vi "Control AlgorithmV3.vi"(5 "Gear (H/L)":bool, 6 "PID Gains":cluster{"P":dbl, "I":dbl, "D":dbl}, 7 "Init":bool, 8 "Motor to Control":u8, 9 "Manual Control":bool, 10 "Wheel Angles":dbl[](array[numeric]), 11 "JoystickIn":i32[](array[slide]) scale=-37626.0..37626.0) -> (2 "Target Angles":dbl[](array[numeric]), 3 "MotorsOut":u16[](array[slide]) scale=0.0..512.0)   [LabVIEW 2013, in "ProcessorHelperFunctions.lvlib"]
uses:
  ProcessorHelperFunctions.lvlib
panel:
  out "AglErr4":dbl
  out "AglErr3":dbl
  out "AglErr2":dbl
  out "AglErr1":dbl
  in  "SteeringAssist4_H":dbl=-0.5 format="%#_13g"
  in  "SteeringAssist3_H":dbl=-0.5 format="%#_13g"
  in  "SteeringAssist2_H":dbl=-0.7 format="%#_13g"
  in  "SteeringAssist1_H":dbl=-0.5 format="%#_13g"
  in  "SteeringAssist4_L":dbl=-0.4 format="%#_13g"
  in  "SteeringAssist3_L":dbl=-0.3 format="%#_13g"
  in  "SteeringAssist2_L":dbl=-0.5 format="%#_13g"
  in  "SteeringAssist1_L":dbl=-0.5 format="%#_13g"
  out "JoystickIn_DB":i32[](array[slide]) scale=-37626.0..37626.0
  out "y":dbl
  out "x":dbl
  out "Point":picture
  out "ReverseDir?4":bool
  out "ReverseDir?3":bool
  out "ReverseDir?2":bool
  out "ReverseDir?1":bool
  out "Radius1":dbl
  out "Radius2":dbl
  out "Radius3":dbl
  out "Radius4":dbl
  in  "RJoyMagGain":dbl=0.6
  in  "LJoyMagGain":dbl=1.0
  out "OldAngle4":dbl
  out "OldAngle3":dbl
  out "OldAngle2":dbl
  out "OldAngle1":dbl
  in  "Yw":dbl=15.5
  in  "Xw":dbl=21.5
  # "Xw is x distance between the\nwheels on the robot"
  # "------------------------------------ LOCAL VARIABLES ---------------------------------------"
  # "Yw is y distance between the\nwheels on the robot"
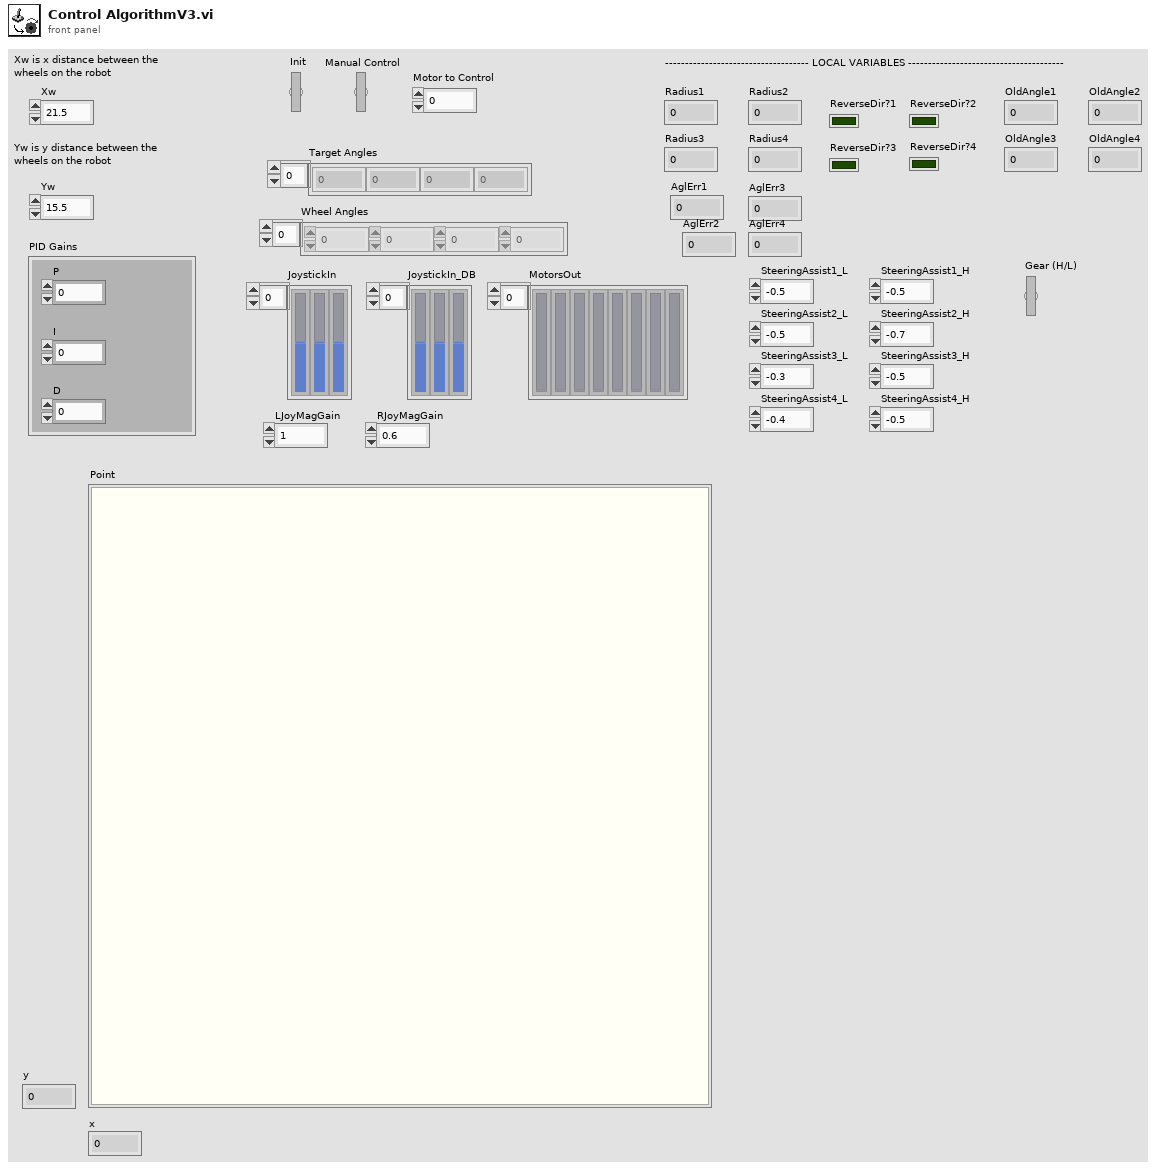
[diagram p1: front panel]
types:
  T1 = cluster{"Width":u16, "Style":enum32{"Solid", "Dash", "Dot", "DashDot", "DashDotDot"}}
  T2 = cluster{"JoystickOut[0]":i32, "JoystickOut[1]":i32, "JoystickOut[2]":i32, "JoystickOut[3]":i32, "JoystickOut[4]":i32, "JoystickOut[5]":i32, "JoystickOut[6]":i32, "JoystickOut[7]":i32, "JoystickOut[8]":i32}
  T3 = cluster{"Wheel Angles[0]":dbl, "Wheel Angles[1]":dbl, "Wheel Angles[2]":dbl, "Wheel Angles[3]":dbl, "Wheel Angles[4]":dbl, "Wheel Angles[5]":dbl, "Wheel Angles[6]":dbl, "Wheel Angles[7]":dbl, "Wheel Angles[8]":dbl}
  T4 = cluster{"[0]":dbl, "[1]":dbl, "[2]":dbl, "[3]":dbl, "[4]":dbl, "[5]":dbl, "[6]":dbl, "[7]":dbl, "[8]":dbl}
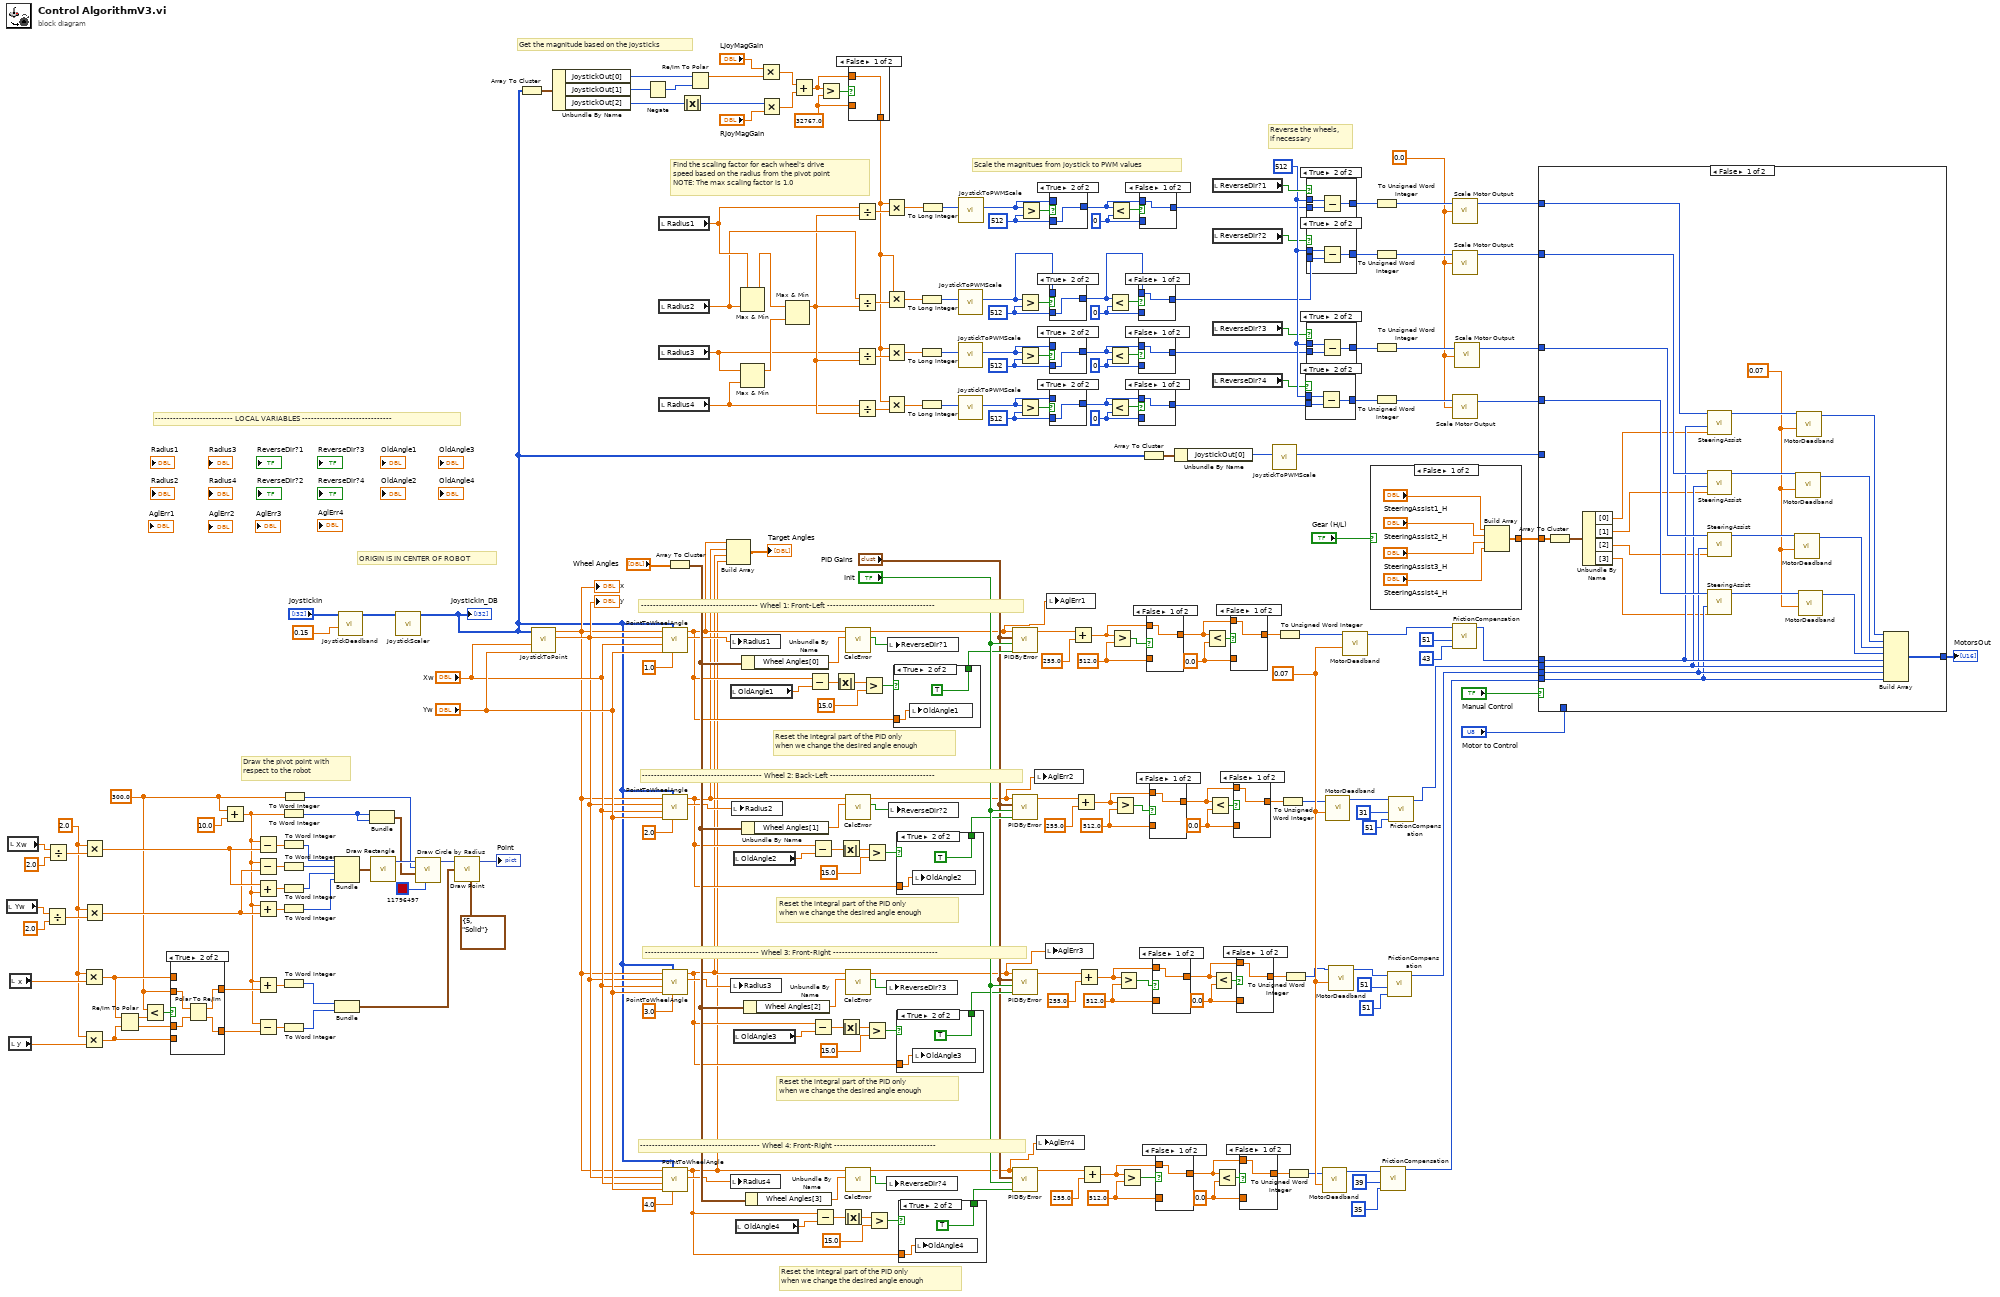
[diagram p0: block diagram]
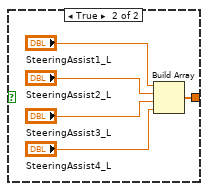
[diagram p2: hidden frame]
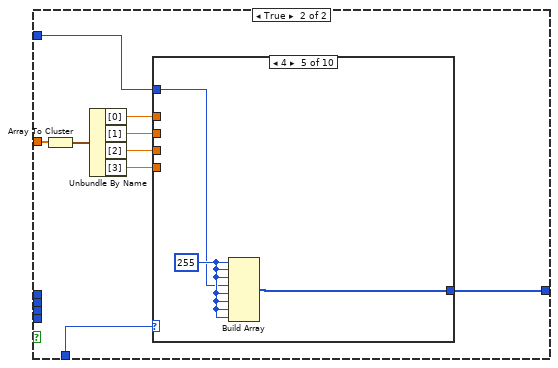
[diagram p17: hidden frame]
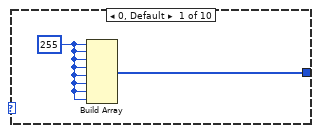
[diagram p18: hidden frame]
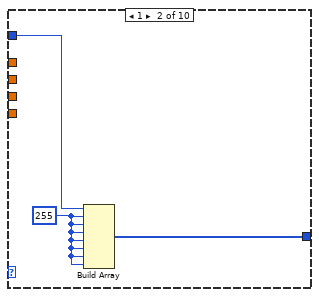
[diagram p19: hidden frame]
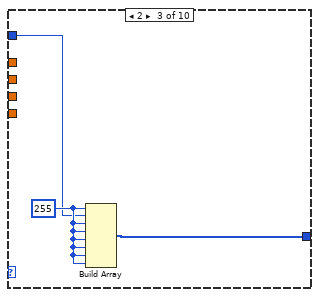
[diagram p20: hidden frame]
diagram:
  w1 = 0.0
  w32 = 0.07 ("DBPercent")
  w42 = 32767.0 ("y")
  w50 = 0 ("y")
  w51 = 512 ("y")
  w61 = 0 ("y")
  w60 = 512 ("y")
  w68 = 0 ("y")
  w69 = 512 ("y")
  w83 = u16 512 ("x")
  w114 = 2.0 ("x")
  w95 = 300.0 ("x")
  w165 = 0 ("y")
  w164 = 512 ("y")
  w184 = 0.0 ("y")
  w182 = 512.0 ("y")
  w190 = 0.0 ("y")
  w192 = 512.0 ("y")
  w200 = 0.0 ("y")
  w198 = 512.0 ("y")
  w205 = 0.0 ("y")
  w207 = 512.0 ("y")
  # "Scale the magnitues from joystick to PWM values"
  # "Get the magnitude based on the joysticks"
  # "Reverse the wheels,\nif necessary"
  # "Draw the pivot point with\nrespect to the robot"
  # "Find the scaling factor for each wheel's drive\nspeed based on the radius from the pivot point\nNOTE: The max scaling factor is 1.0"
  # "Reset the integral part of the PID only\nwhen we change the desired angle enough"
  # "Reset the integral part of the PID only\nwhen we change the desired angle enough"
  # "Reset the integral part of the PID only\nwhen we change the desired angle enough"
  # "Reset the integral part of the PID only\nwhen we change the desired angle enough"
  # "-------------------------- LOCAL VARIABLES ------------------------------"
  # "---------------------------------------- Wheel 4: Front-Right ----------------------------------"
  # "-------------------------------------- Wheel 3: Front-Right -----------------------------------"
  # "---------------------------------------- Wheel 2: Back-Left -----------------------------------"
  # "--------------------------------------- Wheel 1: Front-Left ------------------------------------"
  # "ORIGIN IS IN CENTER OF ROBOT"
  n1 = local read "Yw"() -> (w139:dbl)
  n2 = local read "Xw"() -> (w142:dbl)
  n3 = local read "y"() -> (w115:dbl)
  n4 = local read "x"() -> (w122:dbl)
  n5 = Divide(x=w139, y=2.0) -> (x/y=w119:dbl)
  n6 = Divide(x=w142, y=2.0) -> (x/y=w120:dbl)
  n7 = Multiply(x=w114, y=w122) -> (x*y=w109:dbl)
  n8 = Multiply(x=w114, y=w115) -> (x*y=w108:dbl)
  n9 = Multiply(x=w114, y=w120) -> (x*y=w117:dbl)
  n10 = Multiply(x=w114, y=w119) -> (x*y=w116:dbl)
  n11 = Re/Im To Polar(2:w108, 3:w109) -> (0:w107:dbl, 1:w111:dbl)
  n12 = Less?(x=w95, y=w111) -> (x < y?=w110:bool)
  n13 = case shown="True" w110 {
    tunnel: w109 -> [w251 _]
    tunnel: w108 -> [w250 _]
    tunnel: w95 -> [_ w255]
    tunnel: w107 -> [_ w254]
    tunnel: [w251 w253] -> w105
    tunnel: [w250 w252] -> w106
    frame False {
    }
    frame True {
      n14 = Polar To Re/Im(2:w254, 3:w255) -> (0:w252:dbl, 1:w253:dbl)
    }
  }
  n15 = Add(x=w95, y=10.0) -> (x+y=w94:dbl)
  n16 = Subtract(x=w94, y=w117) -> (x-y=w100:dbl)
  n17 = Subtract(x=w94, y=w116) -> (x-y=w129:dbl)
  n18 = Add(x=w117, y=w94) -> (x+y=w128:dbl)
  n19 = Add(x=w94, y=w116) -> (x+y=w127:dbl)
  n20 = Add(x=w94, y=w105) -> (x+y=w104:dbl)
  n21 = Subtract(x=w94, y=w106) -> (x-y=w103:dbl)
  n22 = To Word Integer(number=w94) -> (16bit integer=w93:i16)
  n23 = To Word Integer(number=w100) -> (16bit integer=w130:i16)
  n24 = To Word Integer(number=w129) -> (16bit integer=w126:i16)
  n25 = To Word Integer(number=w128) -> (16bit integer=w125:i16)
  n26 = To Word Integer(number=w127) -> (16bit integer=w124:i16)
  n27 = To Word Integer(number=w104) -> (16bit integer=w138:i16)
  n28 = To Word Integer(number=w103) -> (16bit integer=w137:i16)
  n29 = To Word Integer(number=w95) -> (16bit integer=w97:i16)
  n30 = Bundle(w130, w126, w125, w124) -> (w123:cluster{i16, i16, i16, i16})  [unwired: 1 in]
  n31 = Bundle(w138, w137) -> (w136:cluster{i16, i16})  [unwired: 1 in]
  n32 = call "JoystickDeadband.vi"("DBPercent"=0.15, "JoystickIn"="JoystickIn") -> ("JoystickOut"=w2:i32[])  [unwired: 9 in]
  n33 = Bundle(w93, w93) -> (w99:cluster{i16, i16})  [unwired: 1 in]
  n34 = call <vilib>:"Draw Rectangle.vi"("rect"=w123) -> ("new picture"=w102:picture)  [unwired: 8 in]
  n35 = call "JoystickScaler.vi"("JoystickIn"=w2) -> ("JoystickOut"=w3:i32[])  [unwired: 10 in]
  "JoystickIn_DB" <- w3
  n36 = call <vilib>:"Draw Circle by Radius.vi"("color(black)"=u32 11796497, "pixel center"=w99, "radius"=w97, "picture"=w102) -> ("new picture"=w101:picture)  [unwired: 7 in]
  n37 = call <vilib>:"Draw Point.vi"("picture"=w101, "point(x,y)"=w136, "pen"=T1 {"Width"=5, "Style"=enum."Solid"}) -> ("new picture"=→"Point":picture)  [unwired: 6 in]
  n38 = Array To Cluster(array=w3) -> (cluster=w176:T2)
  n39 = call "JoystickToPoint.vi"("Yw"="Yw", "Xw"="Xw", "JoystickIn"=w3) -> ("y"=w243:dbl, "x"=w242:dbl)  [unwired: 7 in]
  "x" <- w242
  "y" <- w243
  n40 = Unbundle By Name(w176) -> ("JoystickOut[0]"=w175:i32, "JoystickOut[1]"=w174:i32, "JoystickOut[2]"=w171:i32)
  n41 = Negate(x=w174) -> (-x=w118:i32)
  n42 = local read "Radius1"() -> (w151:dbl)
  n43 = local read "Radius2"() -> (w150:dbl)
  n44 = local read "Radius3"() -> (w148:dbl)
  n45 = local read "Radius4"() -> (w147:dbl)
  n46 = call "PointToWheelAngle.vi"("Wheel Number"=1.0, "JoystickIn"=w3, "Yw"="Yw", "Xw"="Xw", "y"=w243, "x"=w242) -> ("Radius"=w161:dbl, "Desired Angle"=w92:dbl)  [unwired: 4 in]
  n47 = call "PointToWheelAngle.vi"("Wheel Number"=2.0, "JoystickIn"=w3, "Yw"="Yw", "Xw"="Xw", "y"=w243, "x"=w242) -> ("Radius"=w160:dbl, "Desired Angle"=w91:dbl)  [unwired: 4 in]
  n48 = call "PointToWheelAngle.vi"("Wheel Number"=3.0, "JoystickIn"=w3, "Yw"="Yw", "Xw"="Xw", "y"=w243, "x"=w242) -> ("Radius"=w159:dbl, "Desired Angle"=w90:dbl)  [unwired: 4 in]
  n49 = call "PointToWheelAngle.vi"("Wheel Number"=4.0, "JoystickIn"=w3, "Yw"="Yw", "Xw"="Xw", "y"=w243, "x"=w242) -> ("Radius"=w158:dbl, "Desired Angle"=w89:dbl)  [unwired: 4 in]
  n50 = Array To Cluster(array="Wheel Angles") -> (cluster=w240:T3)
  n51 = Absolute Value(x=w171) -> (abs(x)=w45:i32)
  n52 = Re/Im To Polar(2:w118, 3:w175) -> (1:w173:dbl)  [unwired: 1 out]
  n53 = Build Array(w92, w91, w90, w89) -> (→"Target Angles":dbl[])
  n54 = local write "Radius1"(w161) -> ()
  n55 = local read "OldAngle1"() -> (w235:dbl)
  n56 = local write "Radius4"(w158) -> ()
  n57 = local write "Radius3"(w159) -> ()
  n58 = local write "Radius2"(w160) -> ()
  n59 = local read "OldAngle2"() -> (w228:dbl)
  n60 = local read "OldAngle3"() -> (w223:dbl)
  n61 = local read "OldAngle4"() -> (w218:dbl)
  n62 = Max & Min(x=w151, y=w150) -> (max(x,y)=w153:dbl)  [unwired: 1 out]
  n63 = Max & Min(x=w148, y=w147) -> (max(x,y)=w152:dbl)  [unwired: 1 out]
  n64 = Unbundle By Name(w240) -> ("Wheel Angles[0]"=w239:dbl)
  n65 = Unbundle By Name(w240) -> ("Wheel Angles[1]"=w238:dbl)
  n66 = Unbundle By Name(w240) -> ("Wheel Angles[2]"=w237:dbl)
  n67 = Unbundle By Name(w240) -> ("Wheel Angles[3]"=w236:dbl)
  n68 = Multiply(x="LJoyMagGain", y=w173) -> (x*y=w169:dbl)
  n69 = Multiply(x=w45, y="RJoyMagGain") -> (x*y=w168:dbl)
  n70 = Max & Min(x=w153, y=w152) -> (max(x,y)=w149:dbl)  [unwired: 1 out]
  n71 = Add(x=w169, y=w168) -> (x+y=w43:dbl)
  n72 = Subtract(x=w92, y=w235) -> (x-y=w234:dbl)
  n73 = Subtract(x=w91, y=w228) -> (x-y=w227:dbl)
  n74 = Subtract(x=w90, y=w223) -> (x-y=w222:dbl)
  n75 = Subtract(x=w89, y=w218) -> (x-y=w217:dbl)
  n76 = Greater?(x=w43, y=w42) -> (0:w44:bool)
  n77 = Absolute Value(x=w234) -> (abs(x)=w233:dbl)
  n78 = Absolute Value(x=w227) -> (abs(x)=w226:dbl)
  n79 = Absolute Value(x=w222) -> (abs(x)=w221:dbl)
  n80 = Absolute Value(x=w217) -> (abs(x)=w216:dbl)
  n81 = call "CalcError.vi"("Actual Angle"=w239, "Desired Angle"=w92) -> ("ReverseDir?"=w157:bool, "Angle Error"=w15:dbl)  [unwired: 8 in]
  n82 = call "CalcError.vi"("Actual Angle"=w238, "Desired Angle"=w91) -> ("ReverseDir?"=w156:bool, "Angle Error"=w14:dbl)  [unwired: 8 in]
  n83 = call "CalcError.vi"("Actual Angle"=w237, "Desired Angle"=w90) -> ("ReverseDir?"=w155:bool, "Angle Error"=w13:dbl)  [unwired: 8 in]
  n84 = call "CalcError.vi"("Actual Angle"=w236, "Desired Angle"=w89) -> ("ReverseDir?"=w154:bool, "Angle Error"=w12:dbl)  [unwired: 8 in]
  n85 = case shown="False" w44 {
    tunnel: w43 -> [w256 _]
    tunnel: w42 -> [_ w257]
    tunnel: [w256 w257] -> w33
    frame False {
    }
    frame True {
    }
  }
  n86 = Divide(x=w151, y=w149) -> (x/y=w78:dbl)
  n87 = Divide(x=w150, y=w149) -> (x/y=w77:dbl)
  n88 = Divide(x=w148, y=w149) -> (x/y=w76:dbl)
  n89 = Divide(x=w147, y=w149) -> (x/y=w75:dbl)
  n90 = Greater?(x=w233, y=15.0) -> (0:w231:bool)
  n91 = Greater?(x=w226, y=15.0) -> (0:w224:bool)
  n92 = Greater?(x=w221, y=15.0) -> (0:w219:bool)
  n93 = Greater?(x=w216, y=15.0) -> (0:w214:bool)
  n94 = Multiply(x=w33, y=w78) -> (x*y=w74:dbl)
  n95 = Multiply(x=w33, y=w77) -> (x*y=w65:dbl)
  n96 = Multiply(x=w33, y=w76) -> (x*y=w56:dbl)
  n97 = Multiply(x=w33, y=w75) -> (x*y=w47:dbl)
  n98 = local write "ReverseDir?3"(w155) -> ()
  n99 = local write "ReverseDir?4"(w154) -> ()
  n100 = local write "ReverseDir?1"(w157) -> ()
  n101 = local write "ReverseDir?2"(w156) -> ()
  n102 = case shown="True" w231 {
    tunnel: w92 -> [_ w260]
    tunnel: [FALSE ("Reset1") TRUE ("Reset1")] -> w229
    frame False {
    }
    frame True {
      n103 = local write "OldAngle1"(w260) -> ()
    }
  }
  n104 = case shown="True" w224 {
    tunnel: w91 -> [_ w263]
    tunnel: [FALSE ("Reset1") TRUE ("Reset1")] -> w211
    frame False {
    }
    frame True {
      n105 = local write "OldAngle2"(w263) -> ()
    }
  }
  n106 = case shown="True" w219 {
    tunnel: w90 -> [_ w266]
    tunnel: [FALSE ("Reset1") TRUE ("Reset1")] -> w213
    frame False {
    }
    frame True {
      n107 = local write "OldAngle3"(w266) -> ()
    }
  }
  n108 = case shown="True" w214 {
    tunnel: w89 -> [_ w269]
    tunnel: [FALSE ("Reset1") TRUE ("Reset1")] -> w212
    frame False {
    }
    frame True {
      n109 = local write "OldAngle4"(w269) -> ()
    }
  }
  n110 = To Long Integer(number=w65) -> (32bit integer=w66:i32)
  n111 = To Long Integer(number=w56) -> (32bit integer=w63:i32)
  n112 = To Long Integer(number=w47) -> (32bit integer=w48:i32)
  n113 = To Long Integer(number=w74) -> (32bit integer=w167:i32)
  n114 = call "JoystickToPWMScale.vi"("Numeric"=w66) -> ("Numeric 2"=w71:u16)  [unwired: 10 in]
  n115 = call "JoystickToPWMScale.vi"("Numeric"=w63) -> ("Numeric 2"=w58:u16)  [unwired: 10 in]
  n116 = call "JoystickToPWMScale.vi"("Numeric"=w48) -> ("Numeric 2"=w53:u16)  [unwired: 10 in]
  n117 = call "JoystickToPWMScale.vi"("Numeric"=w167) -> ("Numeric 2"=w162:u16)  [unwired: 10 in]
  n118 = call "PIDByError.vi"("Error"=w15, "PID Gains"="PID Gains", "Init"="Init", "Reset"=w229) -> ("Control"=w210:dbl)  [unwired: 6 in]
  n119 = call "PIDByError.vi"("Error"=w14, "PID Gains"="PID Gains", "Init"="Init", "Reset"=w211) -> ("Control"=w195:dbl)  [unwired: 6 in]
  n120 = call "PIDByError.vi"("Error"=w13, "PID Gains"="PID Gains", "Init"="Init", "Reset"=w213) -> ("Control"=w187:dbl)  [unwired: 6 in]
  n121 = call "PIDByError.vi"("Error"=w12, "PID Gains"="PID Gains", "Init"="Init", "Reset"=w212) -> ("Control"=w179:dbl)  [unwired: 6 in]
  n122 = Greater?(x=w71, y=w69) -> (0:w70:bool)
  n123 = Greater?(x=w58, y=w60) -> (0:w59:bool)
  n124 = Greater?(x=w53, y=w51) -> (0:w52:bool)
  n125 = Greater?(x=w162, y=w164) -> (0:w163:bool)
  n126 = local write "AglErr2"(w14) -> ()
  n127 = local write "AglErr4"(w12) -> ()
  n128 = local write "AglErr3"(w13) -> ()
  n129 = local write "AglErr1"(w15) -> ()
  n130 = case shown="True" w70 {
    tunnel: w69 -> [_ w271]
    tunnel: w71 -> [w270 _]
    tunnel: [w270 w271] -> w67
    frame False {
    }
    frame True {
    }
  }
  n131 = case shown="True" w59 {
    tunnel: w60 -> [_ w273]
    tunnel: w58 -> [w272 _]
    tunnel: [w272 w273] -> w62
    frame False {
    }
    frame True {
    }
  }
  n132 = case shown="True" w52 {
    tunnel: w51 -> [_ w275]
    tunnel: w53 -> [w274 _]
    tunnel: [w274 w275] -> w49
    frame False {
    }
    frame True {
    }
  }
  n133 = case shown="True" w163 {
    tunnel: w164 -> [_ w277]
    tunnel: w162 -> [w276 _]
    tunnel: [w276 w277] -> w166
    frame False {
    }
    frame True {
    }
  }
  n134 = Add(x=w210, y=255.0) -> (x+y=w206:dbl)
  n135 = Add(x=w195, y=255.0) -> (x+y=w199:dbl)
  n136 = Add(x=w187, y=255.0) -> (x+y=w191:dbl)
  n137 = Add(x=w179, y=255.0) -> (x+y=w183:dbl)
  n138 = Less?(x=w67, y=w68) -> (x < y?=w72:bool)
  n139 = Less?(x=w62, y=w61) -> (x < y?=w57:bool)
  n140 = Less?(x=w49, y=w50) -> (x < y?=w54:bool)
  n141 = Less?(x=w166, y=w165) -> (x < y?=w131:bool)
  n142 = Greater?(x=w206, y=w207) -> (0:w208:bool)
  n143 = Greater?(x=w199, y=w198) -> (0:w197:bool)
  n144 = Greater?(x=w191, y=w192) -> (0:w193:bool)
  n145 = Greater?(x=w183, y=w182) -> (0:w181:bool)
  n146 = case shown="False" w72 {
    tunnel: w68 -> [_ w279]
    tunnel: w67 -> [w278 _]
    tunnel: [w278 w279] -> w64
    frame False {
    }
    frame True {
    }
  }
  n147 = case shown="False" w57 {
    tunnel: w61 -> [_ w281]
    tunnel: w62 -> [w280 _]
    tunnel: [w280 w281] -> w55
    frame False {
    }
    frame True {
    }
  }
  n148 = case shown="False" w54 {
    tunnel: w50 -> [_ w283]
    tunnel: w49 -> [w282 _]
    tunnel: [w282 w283] -> w46
    frame False {
    }
    frame True {
    }
  }
  n149 = case shown="False" w131 {
    tunnel: w165 -> [_ w285]
    tunnel: w166 -> [w284 _]
    tunnel: [w284 w285] -> w73
    frame False {
    }
    frame True {
    }
  }
  n150 = Array To Cluster(array=w3) -> (cluster=w146:T2)
  n151 = case shown="False" w208 {
    tunnel: w207 -> [_ w287]
    tunnel: w206 -> [w286 _]
    tunnel: [w286 w287] -> w204
    frame False {
    }
    frame True {
    }
  }
  n152 = case shown="False" w197 {
    tunnel: w198 -> [_ w289]
    tunnel: w199 -> [w288 _]
    tunnel: [w288 w289] -> w201
    frame False {
    }
    frame True {
    }
  }
  n153 = case shown="False" w193 {
    tunnel: w192 -> [_ w291]
    tunnel: w191 -> [w290 _]
    tunnel: [w290 w291] -> w189
    frame False {
    }
    frame True {
    }
  }
  n154 = case shown="False" w181 {
    tunnel: w182 -> [_ w293]
    tunnel: w183 -> [w292 _]
    tunnel: [w292 w293] -> w185
    frame False {
    }
    frame True {
    }
  }
  n155 = Unbundle By Name(w146) -> ("JoystickOut[0]"=w145:i32)
  n156 = Less?(x=w204, y=w205) -> (x < y?=w132:bool)
  n157 = Less?(x=w201, y=w200) -> (x < y?=w133:bool)
  n158 = Less?(x=w189, y=w190) -> (x < y?=w134:bool)
  n159 = local read "ReverseDir?1"() -> (w87:bool)
  n160 = local read "ReverseDir?2"() -> (w81:bool)
  n161 = local read "ReverseDir?3"() -> (w80:bool)
  n162 = local read "ReverseDir?4"() -> (w79:bool)
  n163 = Less?(x=w185, y=w184) -> (x < y?=w135:bool)
  n164 = case shown="False" w132 {
    tunnel: w205 -> [_ w295]
    tunnel: w204 -> [w294 _]
    tunnel: [w294 w295] -> w203
    frame False {
    }
    frame True {
    }
  }
  n165 = case shown="False" w133 {
    tunnel: w200 -> [_ w297]
    tunnel: w201 -> [w296 _]
    tunnel: [w296 w297] -> w202
    frame False {
    }
    frame True {
    }
  }
  n166 = case shown="False" w134 {
    tunnel: w190 -> [_ w299]
    tunnel: w189 -> [w298 _]
    tunnel: [w298 w299] -> w188
    frame False {
    }
    frame True {
    }
  }
  n167 = case shown="False" w135 {
    tunnel: w184 -> [_ w301]
    tunnel: w185 -> [w300 _]
    tunnel: [w300 w301] -> w186
    frame False {
    }
    frame True {
    }
  }
  n168 = call "JoystickToPWMScale.vi"("Numeric"=w145) -> ("Numeric 2"=w144:u16)  [unwired: 10 in]
  n169 = To Unsigned Word Integer(number=w203) -> (unsigned 16bit integer=w23:u16)
  n170 = To Unsigned Word Integer(number=w202) -> (unsigned 16bit integer=w21:u16)
  n171 = To Unsigned Word Integer(number=w188) -> (unsigned 16bit integer=w19:u16)
  n172 = To Unsigned Word Integer(number=w186) -> (unsigned 16bit integer=w17:u16)
  n173 = case shown="True" w79 {
    tunnel: w46 -> [w302 w305]
    tunnel: w83 -> [_ w304]
    tunnel: [w302 w303] -> w82
    frame False {
    }
    frame True {
      n174 = Subtract(x=w304, y=w305) -> (x-y=w303:i32)
    }
  }
  n175 = case shown="True" w87 {
    tunnel: w73 -> [w306 w309]
    tunnel: w83 -> [_ w308]
    tunnel: [w306 w307] -> w86
    frame False {
    }
    frame True {
      n176 = Subtract(x=w308, y=w309) -> (x-y=w307:i32)
    }
  }
  n177 = case shown="True" w81 {
    tunnel: w64 -> [w310 w313]
    tunnel: w83 -> [_ w312]
    tunnel: [w310 w311] -> w84
    frame False {
    }
    frame True {
      n178 = Subtract(x=w312, y=w313) -> (x-y=w311:i32)
    }
  }
  n179 = case shown="True" w80 {
    tunnel: w55 -> [w314 w317]
    tunnel: w83 -> [_ w316]
    tunnel: [w314 w315] -> w85
    frame False {
    }
    frame True {
      n180 = Subtract(x=w316, y=w317) -> (x-y=w315:i32)
    }
  }
  n181 = call "MotorDeadband.vi"("DBPercent"=w32, "MotorIn"=w17) -> ("MotorOut"=w16:u16)  [unwired: 9 in]
  n182 = call "MotorDeadband.vi"("DBPercent"=w32, "MotorIn"=w21) -> ("MotorOut"=w20:u16)  [unwired: 9 in]
  n183 = call "MotorDeadband.vi"("DBPercent"=w32, "MotorIn"=w19) -> ("MotorOut"=w18:u16)  [unwired: 9 in]
  n184 = call "MotorDeadband.vi"("DBPercent"=w32, "MotorIn"=w23) -> ("MotorOut"=w22:u16)  [unwired: 9 in]
  n185 = case shown="False" "Gear (H/L)" {
    tunnel: [w318 w323] -> w29
    frame False {
      n186 = Build Array("SteeringAssist1_H", "SteeringAssist2_H", "SteeringAssist3_H", "SteeringAssist4_H") -> (w318:dbl[])
    }
    frame True {
      n187 = Build Array("SteeringAssist1_L", "SteeringAssist2_L", "SteeringAssist3_L", "SteeringAssist4_L") -> (w323:dbl[])
    }
  }
  n188 = To Unsigned Word Integer(number=w86) -> (unsigned 16bit integer=w11:u16)
  n189 = To Unsigned Word Integer(number=w84) -> (unsigned 16bit integer=w10:u16)
  n190 = To Unsigned Word Integer(number=w85) -> (unsigned 16bit integer=w9:u16)
  n191 = To Unsigned Word Integer(number=w82) -> (unsigned 16bit integer=w8:u16)
  n192 = call "FrictionCompensation.vi"("REV Compensation"=u16 35, "FWD Compensation"=u16 39, "Input"=w16) -> ("Output"=w24:u16)  [unwired: 8 in]
  n193 = call "FrictionCompensation.vi"("REV Compensation"=u16 51, "FWD Compensation"=u16 51, "Input"=w18) -> ("Output"=w25:u16)  [unwired: 8 in]
  n194 = call "FrictionCompensation.vi"("REV Compensation"=u16 51, "FWD Compensation"=u16 31, "Input"=w20) -> ("Output"=w26:u16)  [unwired: 8 in]
  n195 = call "FrictionCompensation.vi"("REV Compensation"=u16 43, "FWD Compensation"=u16 51, "Input"=w22) -> ("Output"=w27:u16)  [unwired: 8 in]
  n196 = call "Scale Motor Output.vi"("Error Input"=w1, "Motor Input"=w11) -> ("Output"=w7:u16)  [unwired: 1 in]
  n197 = call "Scale Motor Output.vi"("Error Input"=w1, "Motor Input"=w10) -> ("Output"=w6:u16)  [unwired: 1 in]
  n198 = call "Scale Motor Output.vi"("Error Input"=w1, "Motor Input"=w8) -> ("Output"=w4:u16)  [unwired: 1 in]
  n199 = call "Scale Motor Output.vi"("Error Input"=w1, "Motor Input"=w9) -> ("Output"=w5:u16)  [unwired: 1 in]
  n200 = case shown="False" "Manual Control" {
    tunnel: w27 -> [w346 _]
    tunnel: w26 -> [w345 _]
    tunnel: w25 -> [w344 _]
    tunnel: w24 -> [w343 _]
    tunnel: [w351 w358] -> w30
    tunnel: "Motor to Control" -> [_ w360]
    tunnel: w7 -> [w350 _]
    tunnel: w6 -> [w349 _]
    tunnel: w5 -> [w348 _]
    tunnel: w4 -> [w347 _]
    tunnel: w144 -> [_ w359]
    tunnel: w29 -> [w342 w356]
    frame False {
      w328 = 0.07 ("DBPercent")
      n201 = Array To Cluster(array=w342) -> (cluster=w341:T4)
      n202 = Unbundle By Name(w341) -> ("[0]"=w340:dbl, "[1]"=w339:dbl, "[2]"=w338:dbl, "[3]"=w337:dbl)
      n203 = call "SteeringAssist.vi"("Gain"=w340, "Steering Input"=w346, "Drive Input"=w350) -> ("Drive Output"=w336:u16)  [unwired: 8 in]
      n204 = call "SteeringAssist.vi"("Gain"=w339, "Steering Input"=w345, "Drive Input"=w349) -> ("Drive Output"=w334:u16)  [unwired: 8 in]
      n205 = call "SteeringAssist.vi"("Gain"=w338, "Steering Input"=w344, "Drive Input"=w348) -> ("Drive Output"=w332:u16)  [unwired: 8 in]
      n206 = call "SteeringAssist.vi"("Gain"=w337, "Steering Input"=w343, "Drive Input"=w347) -> ("Drive Output"=w331:u16)  [unwired: 8 in]
      n207 = call "MotorDeadband.vi"("DBPercent"=w328, "MotorIn"=w332) -> ("MotorOut"=w330:u16)  [unwired: 9 in]
      n208 = call "MotorDeadband.vi"("DBPercent"=w328, "MotorIn"=w334) -> ("MotorOut"=w333:u16)  [unwired: 9 in]
      n209 = call "MotorDeadband.vi"("DBPercent"=w328, "MotorIn"=w336) -> ("MotorOut"=w335:u16)  [unwired: 9 in]
      n210 = call "MotorDeadband.vi"("DBPercent"=w328, "MotorIn"=w331) -> ("MotorOut"=w329:u16)  [unwired: 9 in]
      n211 = Build Array(w335, w333, w330, w329, w346, w345, w344, w343) -> (w351:u16[])
    }
    frame True {
      n212 = Array To Cluster(array=w356) -> (cluster=w357:T4)
      n213 = Unbundle By Name(w357) -> ("[0]"=w355:dbl, "[1]"=w354:dbl, "[2]"=w353:dbl, "[3]"=w352:dbl)
      n214 = case shown="4" w360 {
        tunnel: w359 -> [_ w363 w366 w369 w372 w377 w381 w386 w391 w396]
        tunnel: [w362 w364 w367 w370 w373 w379 w384 w389 w394 w397] -> w358
        tunnel: w355 -> [_ _ _ _ _ w378 _ _ _ _]
        tunnel: w354 -> [_ _ _ _ _ _ w383 _ _ _]
        tunnel: w353 -> [_ _ _ _ _ _ _ w388 _ _]
        tunnel: w352 -> [_ _ _ _ _ _ _ _ w393 _]
        frame 0, Default {
          w361 = u16 255
          n215 = Build Array(w361, w361, w361, w361, w361, w361, w361, w361) -> (w362:u16[])
        }
        frame 1 {
          w365 = u16 255
          n216 = Build Array(w363, w365, w365, w365, w365, w365, w365, w365) -> (w364:u16[])
        }
        frame 2 {
          w368 = u16 255
          n217 = Build Array(w368, w366, w368, w368, w368, w368, w368, w368) -> (w367:u16[])
        }
        frame 3 {
          w371 = u16 255
          n218 = Build Array(w371, w371, w369, w371, w371, w371, w371, w371) -> (w370:u16[])
        }
        frame 4 {
          w374 = u16 255
          n219 = Build Array(w374, w374, w374, w372, w374, w374, w374, w374) -> (w373:u16[])
        }
        frame 5 {
          w376 = u16 255
          n220 = call "SteeringAssist.vi"("Gain"=w378, "Steering Input"=w377, "Drive Input"=w376) -> ("Drive Output"=w375:u16)  [unwired: 8 in]
          n221 = Build Array(w375, w376, w376, w376, w377, w376, w376, w376) -> (w379:u16[])
        }
        frame 6 {
          w380 = u16 255
          n222 = call "SteeringAssist.vi"("Gain"=w383, "Steering Input"=w381, "Drive Input"=w380) -> ("Drive Output"=w382:u16)  [unwired: 8 in]
          n223 = Build Array(w380, w382, w380, w380, w380, w381, w380, w380) -> (w384:u16[])
        }
        frame 7 {
          w385 = u16 255
          n224 = call "SteeringAssist.vi"("Gain"=w388, "Steering Input"=w386, "Drive Input"=w385) -> ("Drive Output"=w387:u16)  [unwired: 8 in]
          n225 = Build Array(w385, w385, w387, w385, w385, w385, w386, w385) -> (w389:u16[])
        }
        frame 8 {
          w390 = u16 255
          n226 = call "SteeringAssist.vi"("Gain"=w393, "Steering Input"=w391, "Drive Input"=w390) -> ("Drive Output"=w392:u16)  [unwired: 8 in]
          n227 = Build Array(w390, w390, w390, w392, w390, w390, w390, w391) -> (w394:u16[])
        }
        frame 10 {
          w395 = u16 255
          n228 = Build Array(w396, w396, w396, w396, w395, w395, w395, w395) -> (w397:u16[])
        }
      }
    }
  }
  "MotorsOut" <- w30
